vi "Abort.vi"() -> ()   [LabVIEW 2025]
panel:
  in  "Abort":bool
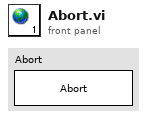
[diagram p1: front panel]
diagram:
